vi "Configure Dialog.vi"(8 "error in (no error)":errorcluster, 11 "Create SV Msg.lvclass":refnum<class "Create SV Msg.lvclass">) -> (0 "error out":errorcluster, 2 "Ok?":bool, 3 "Create SV Msg.lvclass":refnum<class "Create SV Msg.lvclass">)   [LabVIEW 2015, in "CS++DSCManager.lvlib" / "Create SV Msg.lvclass"]
doc: "This overrides of this dynamic dispatch VI open the frontpanel to set derived message attributes."
uses:
  Create SV Msg.lvclass
  Create SV Msg.lvclass/Create SV Msg.ctl
panel:
  in  "custom control":variant
  in  "data type":T1(ring)
  in  "Mode":u16
  in  "shared variable name":string
  in  "process name":string
  in  "Cancel Button":bool
  in  "OK Button":bool
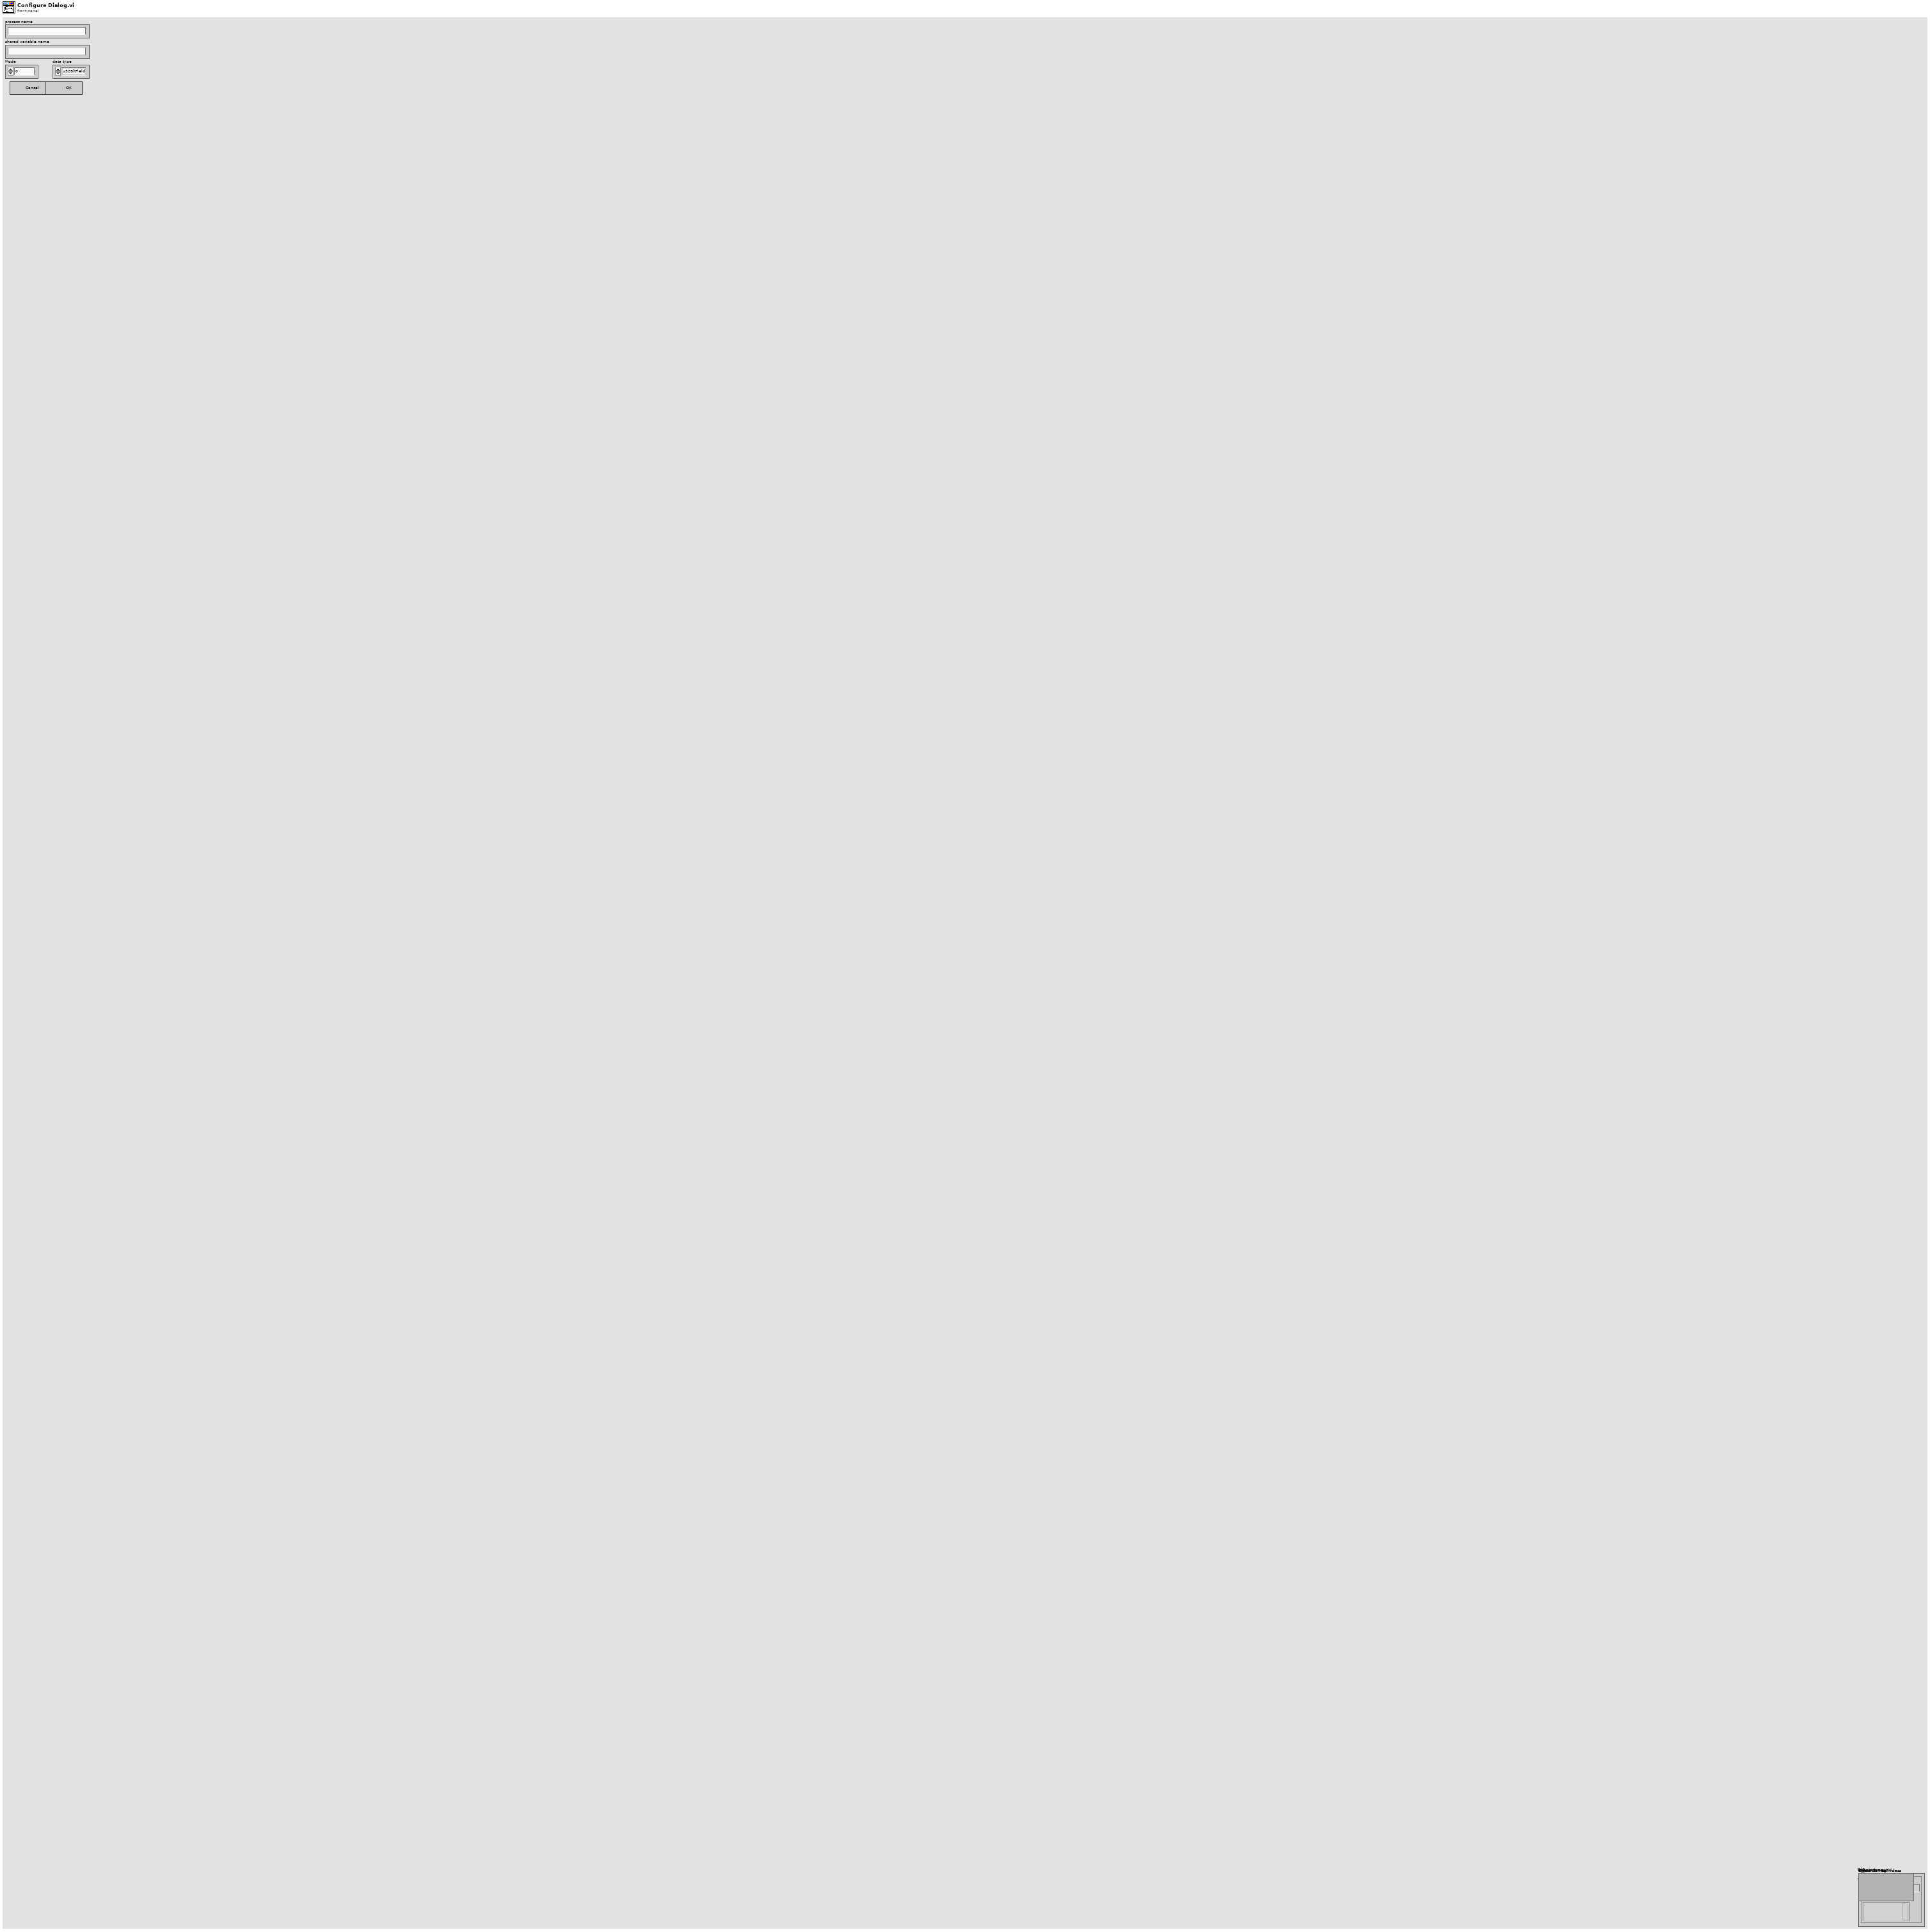
[diagram p1: front panel]
types:
  T1 = enum32{"u32BitField", "bool", "double", "string", "int8", "uint8", "int16", "uint16", "int32", "uint32", "int64", "uint64", "single", "double waveform", "int16 waveform", "array of boolean", "array of int8", "array of uint8", "array of int16", "array of uint16", "array of int32", "array of uint32", "array of int64", "array of uint64", "array of single", "array of double", "array of double waveform", "array of int16 waveform", "array of string", "variant", "timestamp", "fixed point", "custom"}
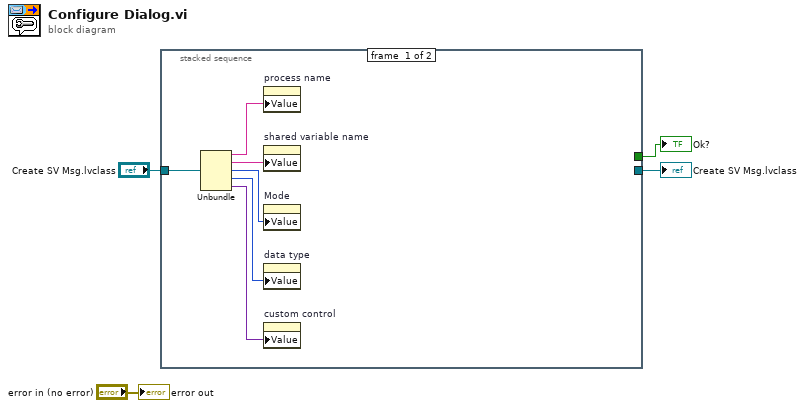
[diagram p0: block diagram]
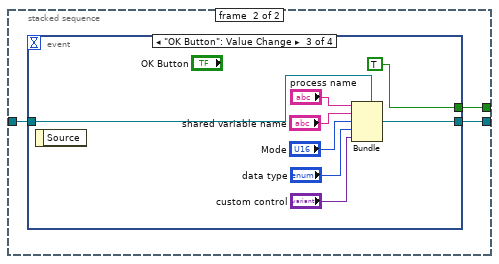
[diagram p2: hidden frame]
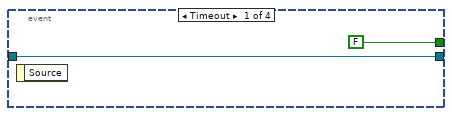
[diagram p3: hidden frame]
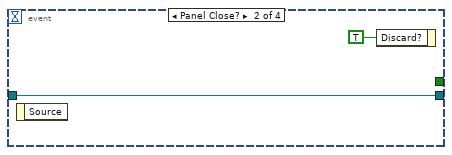
[diagram p4: hidden frame]
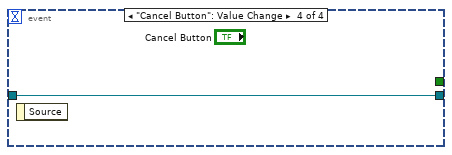
[diagram p5: hidden frame]
diagram:
  n1 = stacked-sequence {
    tunnel: [_ w13] -> w3
    tunnel: [_ w12] -> w2
    tunnel: "Create SV Msg.lvclass" -> [w10 w11]
    frame #0 {
      n2 = Unbundle ("Seq0Unbundler")(w10) -> (w9:string, w8:string, w7:u16, w6:T1, w5:variant)
      n3 = property on="process name" class="Str"("Value"=w9) -> ()  [unwired: 2 in, 2 out]
      n4 = property on="shared variable name" class="Str"("Value"=w8) -> ()  [unwired: 2 in, 2 out]
      n5 = property on="Mode" class="DigNum (strict)"("Value"=w7) -> ()  [unwired: 2 in, 2 out]
      n6 = property on="data type" class="Enum (strict)"("Value"=w6) -> ()  [unwired: 2 in, 2 out]
      n7 = property on="custom control" class="LVVar"("Value"=w5) -> ()  [unwired: 2 in, 2 out]
    }
    frame #1 {
      n8 = event shown="[2] \"OK Button\": Value Change" {
        selector: _ -> [_ _ _ _]
        dyn-events: _ -> [_ _ _ _]
        timeout: _ -> [_ _ _ _]
        tunnel: [w14 w16 w23 w26] -> w12
        tunnel: w11 -> [w14 w16 w25 w26]
        tunnel: [FALSE _ TRUE _] -> w13
        event Timeout {
          n9 = event-data() -> ()  [unwired: 1 in, 1 out]
        }
        event Panel Close? {
          n10 = event-data() -> ()  [unwired: 1 in, 1 out]
          n11 = event-data ("Event Filter Node")("Discard?"=TRUE) -> ()  [unwired: 1 in, 1 out]
        }
        event "OK Button": Value Change {
          n12 = event-data() -> ()  [unwired: 1 in, 1 out]
          n13 = Bundle ("Main-Bundler")(cluster=w25, "process name", "shared variable name", "Mode", "data type", "custom control") -> (w23:refnum<class "Create SV Msg.lvclass">)
        }
        event "Cancel Button": Value Change {
          n14 = event-data() -> ()  [unwired: 1 in, 1 out]
        }
      }
    }
  }
  "Ok?" <- w3
  "Create SV Msg.lvclass" <- w2
  "error out" <- "error in (no error)"
